vi "V50 Report Part 1 (SubVI).vi"(0 "NI_report in":refnum<class "NI_report.lvclass">, 5 "SampleID":string, 11 "error in (no error)":errorcluster) -> (4 "NI_report out":refnum<class "NI_report.lvclass">, 15 "error out":errorcluster)   [LabVIEW 2015]
uses:
  <vilib>/Utility/NIReport.llb/NI_report.lvclass
  <vilib>/Utility/NIReport.llb/Append Report Text (str wrap).vi
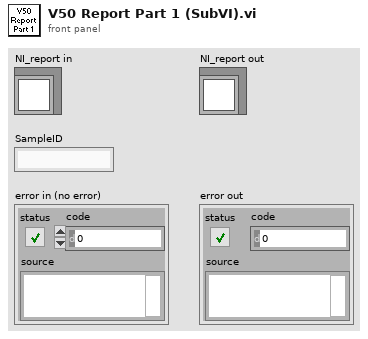
[diagram p1: front panel]
types:
  T1 = cluster{"position (excel)":cluster{"row":i32, "column":i32}, "name (excel)":string, "bookmark (word)":string}
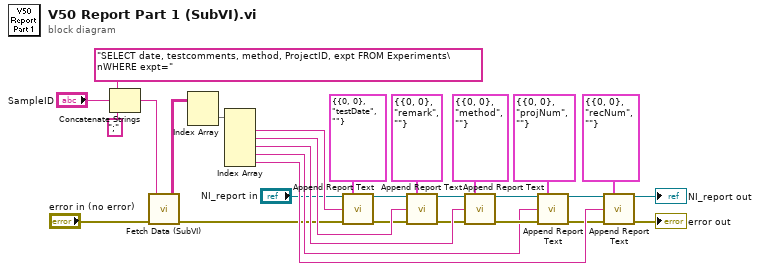
[diagram p0: block diagram]
diagram:
  n1 = Concatenate Strings("SELECT date, testcomments, method, ProjectID, expt FROM Experiments\nWHERE expt=" ("query string"), "SampleID", ";" ("string")) -> (w8:string)
  n2 = call "Fetch Data (SubVI).vi"("error IN"="error in (no error)", "query string"=w8) -> ("error OUT"=w1:errorcluster, "recordset data"=w9:string[][])  [unwired: 4 out]
  n3 = Index Array(array=w9) -> (element=w10:string[])  [unwired: 2 in]
  n4 = Index Array(array=w10) -> (element #1=w11:string, element #2=w14:string, element #3=w22:string, element #4=w23:string, element #5=w24:string)  [unwired: 5 in]
  n5 = call-poly <vilib>:"Append Report Text.vi"("report in"="NI_report in", "MS Office parameters"=T1 {"position (excel)"={"row"=0, "column"=0}, "name (excel)"="testDate", "bookmark (word)"=""}, "text"=w11, "error in (no error)"=w1) -> ("report out"=w5:refnum<class "NI_report.lvclass">, "error out"=w4:errorcluster)  [unwired: 8 in, 2 out]
  n6 = call-poly <vilib>:"Append Report Text.vi"("report in"=w5, "MS Office parameters"=T1 {"position (excel)"={"row"=0, "column"=0}, "name (excel)"="remark", "bookmark (word)"=""}, "text"=w14, "error in (no error)"=w4) -> ("report out"=w16:refnum<class "NI_report.lvclass">, "error out"=w17:errorcluster)  [unwired: 8 in, 2 out]
  n7 = call-poly <vilib>:"Append Report Text.vi"("report in"=w16, "MS Office parameters"=T1 {"position (excel)"={"row"=0, "column"=0}, "name (excel)"="method", "bookmark (word)"=""}, "text"=w22, "error in (no error)"=w17) -> ("report out"=w27:refnum<class "NI_report.lvclass">, "error out"=w28:errorcluster)  [unwired: 8 in, 2 out]
  n8 = call-poly <vilib>:"Append Report Text.vi"("report in"=w27, "MS Office parameters"=T1 {"position (excel)"={"row"=0, "column"=0}, "name (excel)"="projNum", "bookmark (word)"=""}, "text"=w23, "error in (no error)"=w28) -> ("report out"=w20:refnum<class "NI_report.lvclass">, "error out"=w21:errorcluster)  [unwired: 8 in, 2 out]
  n9 = call-poly <vilib>:"Append Report Text.vi"("report in"=w20, "MS Office parameters"=T1 {"position (excel)"={"row"=0, "column"=0}, "name (excel)"="recNum", "bookmark (word)"=""}, "text"=w24, "error in (no error)"=w21) -> ("report out"=→"NI_report out":refnum<class "NI_report.lvclass">, "error out"=→"error out":errorcluster)  [unwired: 8 in, 2 out]
